vi "Set UI Theme.vi"(7 "theme":T2=enum."edit buttons disable state", 8 "error in (no error)":errorcluster, 9 "flags":T1, 10 "global scope?":T3=enum."global", 11 "control references":T4) -> (0 "error out":errorcluster)   [LabVIEW 2017]
uses:
  Controls/Error Codes List Window References.ctl
  Error List/Scope.ctl
  Controls/Themes.ctl
  Controls/Flags.ctl
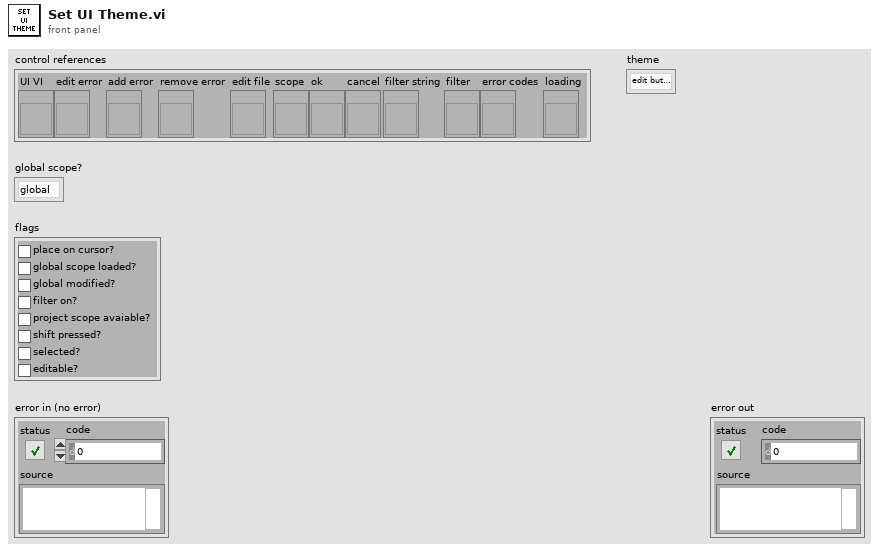
[diagram p1: front panel]
types:
  T1 = typedef "Flags.ctl" = cluster{"place on cursor?":bool, "global scope loaded?":bool, "global modified?":bool, "filter on?":bool, "project scope avaiable?":bool, "shift pressed?":bool, "selected?":bool, "editable?":bool}
  T2 = typedef "Themes.ctl" = enum16{"init", "edit buttons disable state", "loading on", "loading off", "scope name"}
  T3 = typedef "Scope.ctl" = enum16{"project", "global"}
  T4 = typedef "Error Codes List Window References.ctl" = cluster{"UI VI":refnum<vi>, "edit error":refnum<vi>, "add error":refnum<vi>, "remove error":refnum<vi>, "edit file":refnum<vi>, "scope":refnum<vi>, "ok":refnum<vi>, "cancel":refnum<vi>, "filter string":refnum<vi>, "filter":refnum<vi>, "error codes":refnum<vi>, "loading":refnum<vi>}
  T5 = enum8{"Enabled", "Disabled", "Disabled and Grayed Out"}
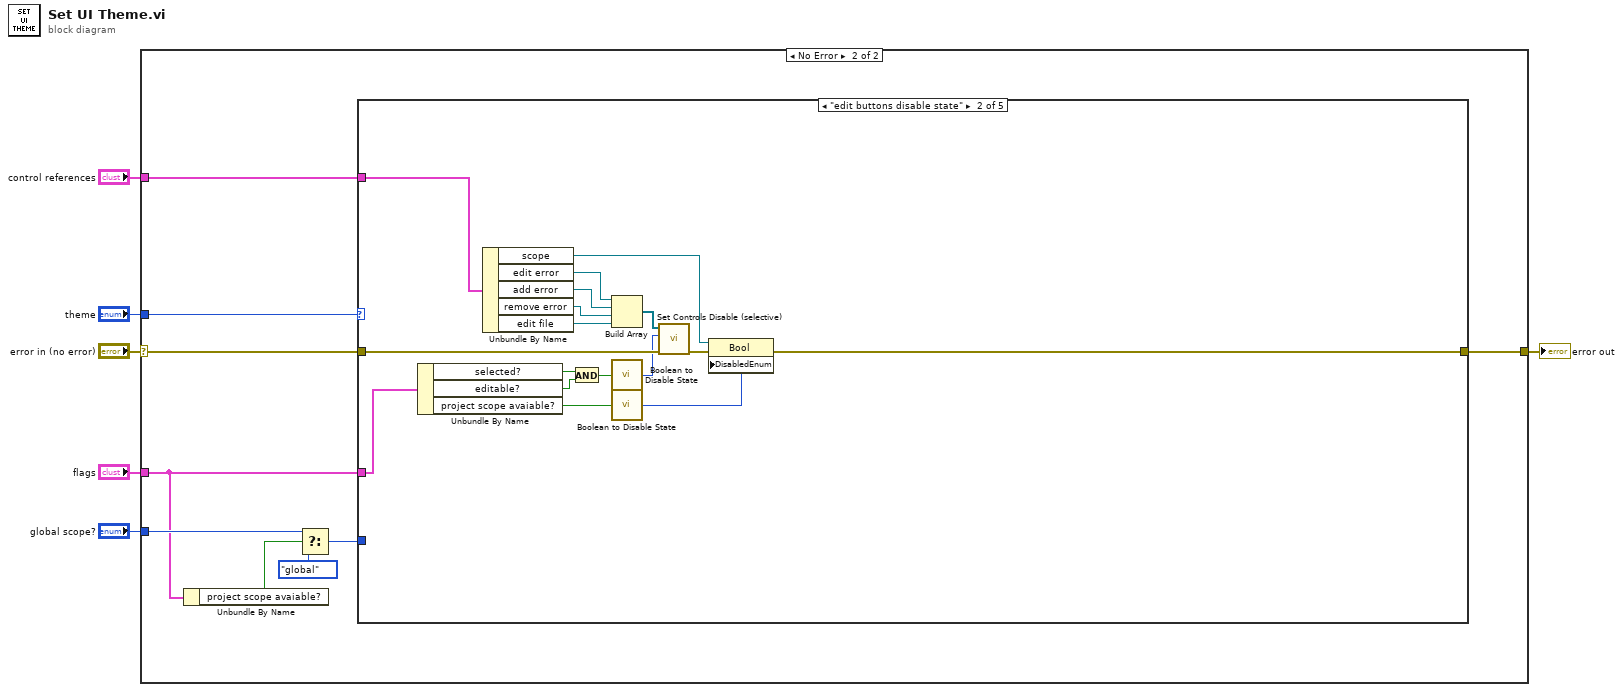
[diagram p0: block diagram]
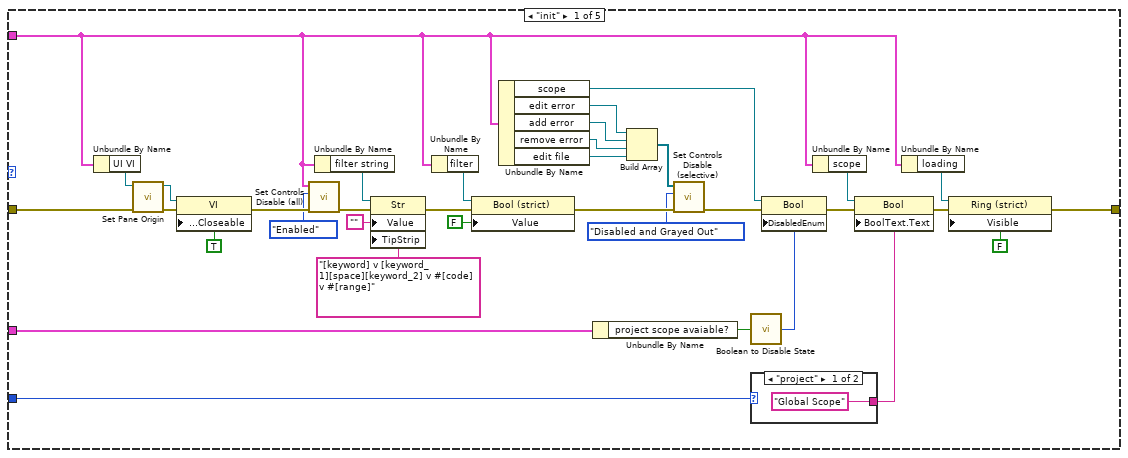
[diagram p3: hidden frame]
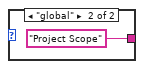
[diagram p4: hidden frame]
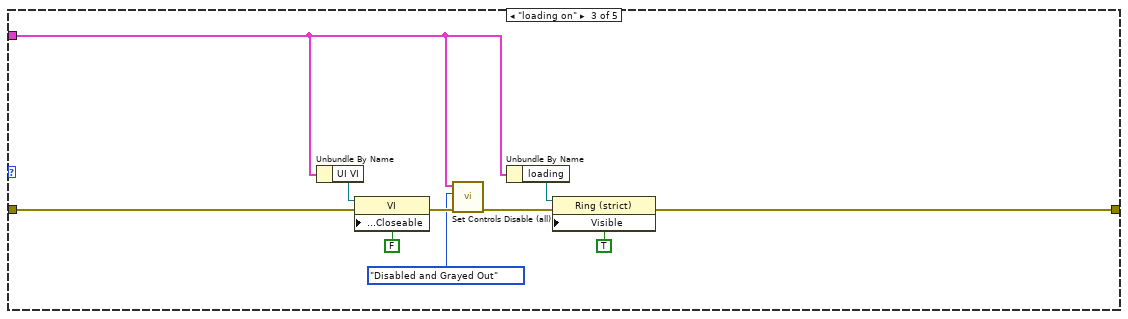
[diagram p5: hidden frame]
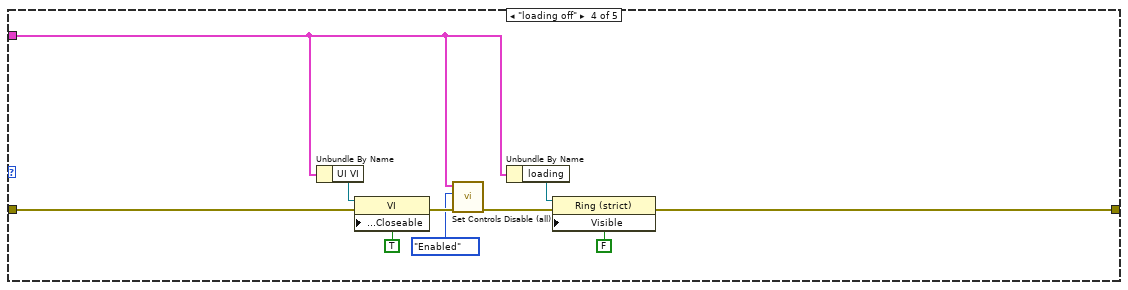
[diagram p6: hidden frame]
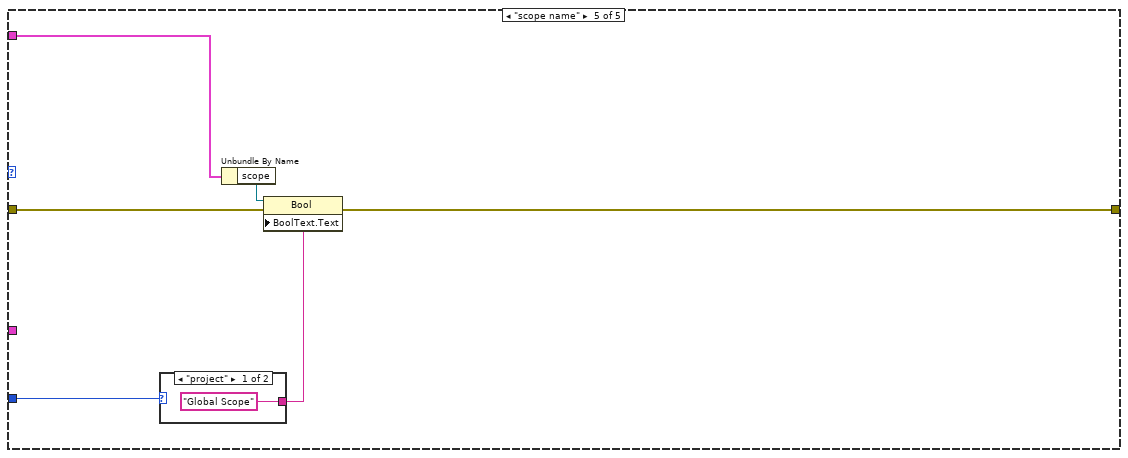
[diagram p7: hidden frame]
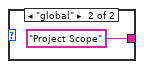
[diagram p8: hidden frame]
diagram:
  n1 = case shown="No Error" "error in (no error)" {
    selector: "error in (no error)" -> [w7 w14]
    tunnel: "global scope?" -> [_ w12]
    tunnel: "control references" -> [_ w16]
    tunnel: [w7 w15] -> w5
    tunnel: "theme" -> [_ w13]
    tunnel: "flags" -> [_ w9]
    frame Error {
    }
    frame No Error {
      n2 = Unbundle By Name(w9) -> ("project scope avaiable?"=w8:bool)
      n3 = Select(t=w12, s=w8, f=Scope."global") -> (s? t:f=w10:T3)
      n4 = case shown="\"edit buttons disable state\"" w13 {
        tunnel: w16 -> [w20 w64 w75 w85 w93]
        tunnel: w10 -> [w44 _ _ _ w92]
        tunnel: w14 -> [w35 w60 w72 w82 w94]
        tunnel: [w19 w62 w71 w81 w95] -> w15
        tunnel: w9 -> [w22 w59 _ _ _]
        frame "init" {
          n5 = Unbundle By Name(w20) -> ("UI VI"=w34:refnum<vi>)
          n6 = call "Set Pane Origin.vi"("error in (no error)"=w35, "VI (caller)"=w34) -> ("error out"=w33:errorcluster, "VI dup"=w32:refnum<vi>)  [unwired: 8 in]
          n7 = property class="VI"(reference=w32, error in=w33, "Front Panel.Closeable"=TRUE ("Front Panel Window:Closeable")) -> (error out=w50:errorcluster)  [unwired: 1 out]
          n8 = call "Set Controls Disable (all).vi"("error in (no error)"=w50, "disable state"=T5."Enabled" ("Disabled"), "control references"=w20) -> ("error out"=w31:errorcluster)  [unwired: 8 in]
          n9 = Unbundle By Name(w20) -> ("filter string"=w27:refnum<vi>)
          n10 = property on="Property Node" class="Str"(reference=w27, error in=w31, "Value"="", "TipStrip"="[keyword] v [keyword_1][space][keyword_2] v #[code] v #[range]" ("Tip Strip")) -> (error out=w47:errorcluster)  [unwired: 1 out]
          n11 = Unbundle By Name(w20) -> ("filter"=w26:refnum<vi>)
          n12 = property class="Bool (strict)"(reference=w26, error in=w47, "Value"=FALSE) -> (error out=w51:errorcluster)  [unwired: 1 out]
          n13 = Unbundle By Name(w20) -> ("scope"=w36:refnum<vi>, "edit error"=w42:refnum<vi>, "add error"=w41:refnum<vi>, "remove error"=w40:refnum<vi>, "edit file"=w39:refnum<vi>)
          n14 = Unbundle By Name(w22) -> ("project scope avaiable?"=w18:bool)
          n15 = Build Array(w42, w41, w40, w39) -> (w38:refnum<vi>[])
          n16 = call "Set Controls Disable (selective).vi"("error in (no error)"=w51, "disabled"=T5."Disabled and Grayed Out" ("Disabled"), "ctrls"=w38) -> ("error out"=w23:errorcluster)  [unwired: 7 in, 1 out]
          n17 = call "Boolean to Disable State.vi"("enable?"=w18) -> ("disable state"=w17:T5)
          n18 = case shown="\"project\"" w44 {
            tunnel: ["Global Scope" "Project Scope"] -> w43
            frame "project" {
            }
            frame "global" {
            }
          }
          n19 = property on="Property Node" class="Bool"(reference=w36, error in=w23, "DisabledEnum"=w17) -> (error out=w21:errorcluster)  [unwired: 1 out]
          n20 = Unbundle By Name(w20) -> ("scope"=w25:refnum<vi>)
          n21 = property on="Property Node" class="Bool"(reference=w25, error in=w21, "BoolText.Text"=w43) -> (error out=w28:errorcluster)  [unwired: 1 out]
          n22 = Unbundle By Name(w20) -> ("loading"=w24:refnum<vi>)
          n23 = property on="Property Node" class="Ring (strict)"(reference=w24, error in=w28, "Visible"=FALSE) -> (error out=w19:errorcluster)  [unwired: 1 out]
        }
        frame "edit buttons disable state" {
          n24 = Unbundle By Name(w59) -> ("selected?"=w58:bool, "editable?"=w57:bool, "project scope avaiable?"=w54:bool)
          n25 = Unbundle By Name(w64) -> ("scope"=w65:refnum<vi>, "edit error"=w70:refnum<vi>, "add error"=w69:refnum<vi>, "remove error"=w68:refnum<vi>, "edit file"=w67:refnum<vi>)
          n26 = And(x=w58, y=w57) -> (x .and. y?=w63:bool)
          n27 = Build Array(w70, w69, w68, w67) -> (w66:refnum<vi>[])
          n28 = call "Boolean to Disable State.vi"("enable?"=w63) -> ("disable state"=w56:T5)
          n29 = call "Boolean to Disable State.vi"("enable?"=w54) -> ("disable state"=w55:T5)
          n30 = call "Set Controls Disable (selective).vi"("error in (no error)"=w60, "disabled"=w56, "ctrls"=w66) -> ("error out"=w61:errorcluster)  [unwired: 7 in, 1 out]
          n31 = property on="Property Node" class="Bool"(reference=w65, error in=w61, "DisabledEnum"=w55) -> (error out=w62:errorcluster)  [unwired: 1 out]
        }
        frame "loading on" {
          n32 = Unbundle By Name(w75) -> ("UI VI"=w76:refnum<vi>)
          n33 = property class="VI"(reference=w76, error in=w72, "Front Panel.Closeable"=FALSE ("Front Panel Window:Closeable")) -> (error out=w80:errorcluster)  [unwired: 1 out]
          n34 = call "Set Controls Disable (all).vi"("error in (no error)"=w80, "disable state"=T5."Disabled and Grayed Out" ("Disabled"), "control references"=w75) -> ("error out"=w77:errorcluster)  [unwired: 8 in]
          n35 = Unbundle By Name(w75) -> ("loading"=w74:refnum<vi>)
          n36 = property class="Ring (strict)"(reference=w74, error in=w77, "Visible"=TRUE) -> (error out=w71:errorcluster)  [unwired: 1 out]
        }
        frame "loading off" {
          n37 = Unbundle By Name(w85) -> ("UI VI"=w86:refnum<vi>)
          n38 = property class="VI"(reference=w86, error in=w82, "Front Panel.Closeable"=TRUE ("Front Panel Window:Closeable")) -> (error out=w90:errorcluster)  [unwired: 1 out]
          n39 = call "Set Controls Disable (all).vi"("error in (no error)"=w90, "disable state"=T5."Enabled" ("Disabled"), "control references"=w85) -> ("error out"=w87:errorcluster)  [unwired: 8 in]
          n40 = Unbundle By Name(w85) -> ("loading"=w84:refnum<vi>)
          n41 = property class="Ring (strict)"(reference=w84, error in=w87, "Visible"=FALSE) -> (error out=w81:errorcluster)  [unwired: 1 out]
        }
        frame "scope name" {
          n42 = case shown="\"project\"" w92 {
            tunnel: ["Global Scope" "Project Scope"] -> w91
            frame "project" {
            }
            frame "global" {
            }
          }
          n43 = Unbundle By Name(w93) -> ("scope"=w96:refnum<vi>)
          n44 = property on="Property Node" class="Bool"(reference=w96, error in=w94, "BoolText.Text"=w91) -> (error out=w95:errorcluster)  [unwired: 1 out]
        }
      }
    }
  }
  "error out" <- w5
